vi "Variant to XY-Data.vi"(2 "error in (no error)":errorcluster, 3 "Value in":variant) -> (0 "error out":errorcluster, 1 "Value out":cluster{"X":dbl[], "Y":dbl[]}[](array[cluster]))   [LabVIEW 2016, in "graph_utilities.lvclass"]
uses:
  graph_utilities.lvclass
  <vilib>/Utility/Data Type/NI_Data Type.lvlib
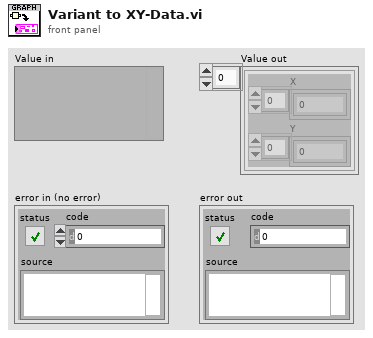
[diagram p1: front panel]
types:
  T1 = typedef "NI_Data Type.lvlib/Data Type.ctl" = enum8{"Invalid Type", "Void", "I8", "I16", "I32", "I64", "U8", "U16", "U32", "U64", "Single Float", "Double Float", "Extended Float", "Single Complex", "Double Complex", "Extended Complex", "Enum U8", "Enum U16", "Enum U32", "Enum U64", "Single Float With Unit", "Double Float With Unit", "Extended Float With Unit", "Single Complex with Unit", "Double Complex with Unit", "Extended Complex with Unit", "Boolean", "String", "Path", "Picture", "Tag", "Array", "Cluster", "Variant", "LV Variant", "Waveform", "Timestamp", "Digital Waveform", "Digital Data", "ExpressData", "Refnum", "External Data", "VI", "Poly VI", "LabVIEW Class Instance", "Fixed Point"}
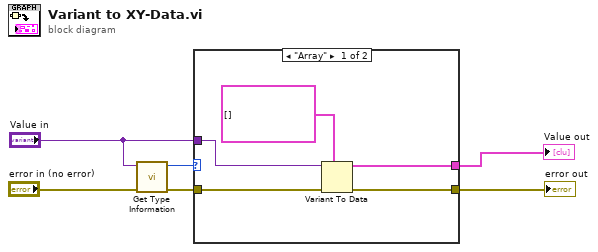
[diagram p0: block diagram]
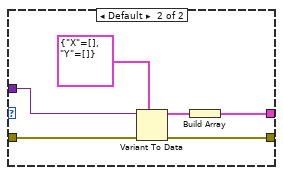
[diagram p2: hidden frame]
diagram:
  n1 = call <vilib>:"Get Type Information.vi"("error in (no error)"="error in (no error)", "Variant"="Value in") -> ("error out"=w3:errorcluster, "Type"=w1:T1)  [unwired: 5 in, 3 out]
  n2 = case shown="\"Array\"" w1 {
    tunnel: [w11 w12] -> w6
    tunnel: [w10 w16] -> w5
    tunnel: w3 -> [w9 w15]
    tunnel: "Value in" -> [w7 w14]
    frame "Array" {
      n3 = Variant To Data(error in=w9, type=cluster{"X":dbl[], "Y":dbl[]}[] [] ("Value"), Variant=w7) -> (data=w11:cluster{"X":dbl[], "Y":dbl[]}[], error out=w10:errorcluster)
    }
    frame Default {
      n4 = Variant To Data(error in=w15, type=cluster{"X":dbl[], "Y":dbl[]} {"X"=[], "Y"=[]}, Variant=w14) -> (data=w17:cluster{"X":dbl[], "Y":dbl[]}, error out=w16:errorcluster)
      n5 = Build Array(w17) -> (w12:cluster{"X":dbl[], "Y":dbl[]}[])
    }
  }
  "Value out" <- w6
  "error out" <- w5
